vi "Reply Table Object.vi"(8 "error in (no error)":errorcluster, 11 "Form Server Messages in":refnum<class "Form Server Messages.lvclass">) -> (0 "error out":errorcluster, 2 "Table":refnum<class "Basic Table.lvclass">, 3 "Form Server Messages out":refnum<class "Form Server Messages.lvclass">)   [LabVIEW 2020]
uses:
  Form Server Messages.lvclass
  Database OOP/Table Libraries/Basic Table/Basic Table Class/Basic Table.lvclass
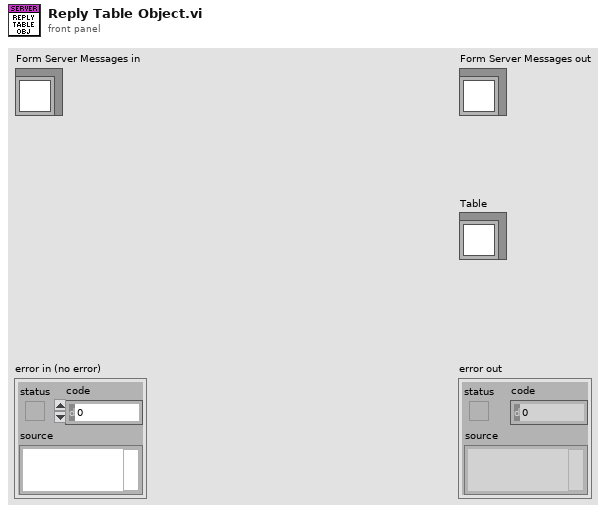
[diagram p1: front panel]
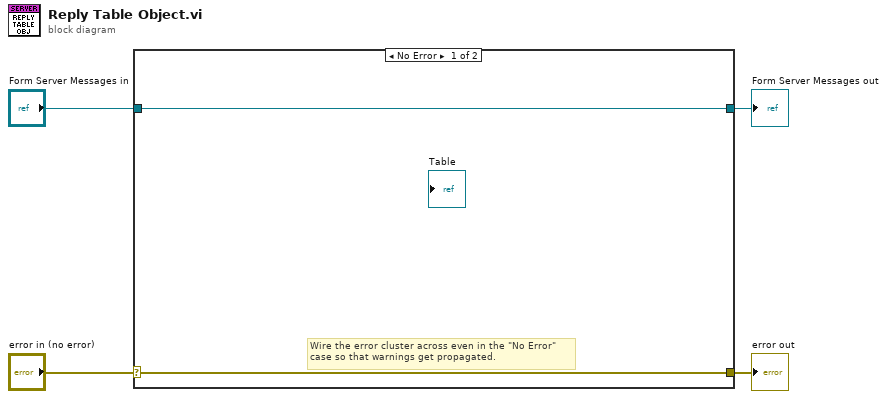
[diagram p0: block diagram]
diagram:
  n1 = case shown="No Error" "error in (no error)" {
    selector: "error in (no error)" -> [w5 w8]
    tunnel: [w5 w8] -> w3
    tunnel: [w6 w7] -> w1
    tunnel: "Form Server Messages in" -> [w6 w7]
    frame No Error {
      # "Wire the error cluster across even in the \"No Error\"\ncase so that warnings get propagated."
    }
    frame Error {
    }
  }
  "error out" <- w3
  "Form Server Messages out" <- w1
